vi "Get Message Definition.vi"(8 "error in":errorcluster, 10 "message name":string, 11 "port in":T6 format="%.0x") -> (0 "error out":errorcluster, 2 "message configuration":T1={"name"="", "message type"="BC to RT", "endpoint Tx"={"terminal address"=0, "subaddress"=0}, "endpoint Rx"={"terminal address"=0, "subaddress"=0}, "create timestamp channel"=FALSE, "mode code"=0, "number of words"=0, "parameters"=[]}, 3 "port out":T6 format="%.0x")   [LabVIEW 2020, in "Ballard MIL-STD-1553 Scripting.lvlib"]
uses:
  Ballard MIL-STD-1553 Scripting.lvlib
  <vilib>/NI VeriStand/Custom Device API/Custom Device Item Ref.ctl
  Shared/Message Definition.ctl
  Shared/Message Type.ctl
  Shared/Terminal Endpoint.ctl
  Shared/Address.ctl
  Shared/Parameter Definition.ctl
  Shared/Direction.ctl
  <vilib>/NI VeriStand/Custom Device API/Custom Device API.lvlib
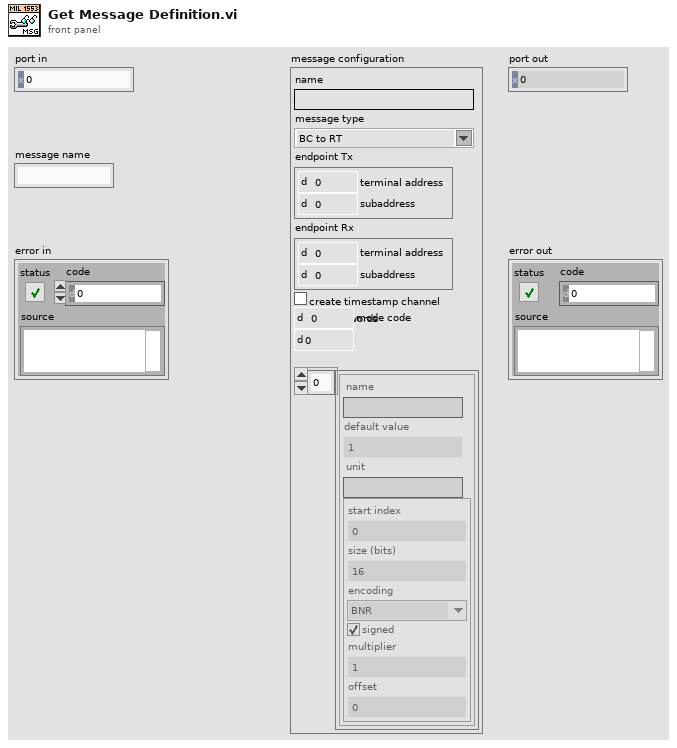
[diagram p1: front panel]
types:
  T1 = typedef "Message Definition.ctl" = cluster{"name":string, "message type":T2, "endpoint Tx":T3, "endpoint Rx":T3, "create timestamp channel":bool, "mode code":u16, "number of words":u16, "parameters":cluster{"name":string, "default value":dbl, "unit":string, "parameter definition":T5}[]}
  T2 = typedef "Message Type.ctl" = string
  T3 = typedef "Terminal Endpoint.ctl" = cluster{"terminal address":T4, "subaddress":T4}
  T4 = typedef "Address.ctl" = u16
  T5 = typedef "Parameter Definition.ctl" = cluster{"start index":i32, "size (bits)":i32, "encoding":enum16{"BNR", "BCD", "Discrete"}, "signed":bool, "multiplier":dbl, "offset":dbl}
  T6 = typedef "Custom Device API.lvlib/Custom Device Item Ref.ctl" = u64
  T7 = typedef "Direction.ctl" = enum16{"Rx", "Tx"}
  T8 = cluster{"name":string, "default value":dbl, "unit":string, "parameter definition":T5}
  T9 = typedef "Custom Device API.lvlib/Custom Device Channel.ctl" = cluster{"Type":T10, "Units":string, "Default Value":dbl, "Faultable":bool, "Scalable":bool}
  T10 = typedef "Custom Device API.lvlib/Custom Device Channel Type.ctl" = enum16{"Input", "Output"}
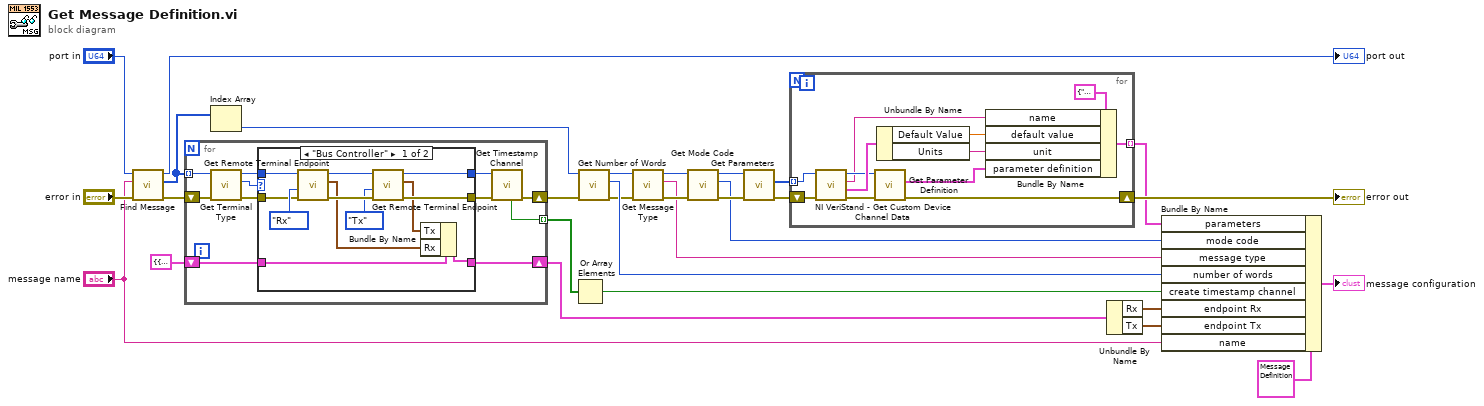
[diagram p0: block diagram]
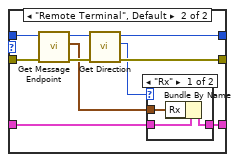
[diagram p2: hidden frame]
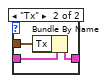
[diagram p3: hidden frame]
diagram:
  n1 = call "Find Message.vi"("error in"="error in", "message name"="message name", "port in"="port in") -> ("error out"=w28:errorcluster, "message refs"=w29:T6[], "port out"=→"port out":T6)  [unwired: 5 in, 1 out]
  n2 = for {
    shift-right: [w39] -> w11
    shift-left: w28 -> [w33]
    tunnel: w29 -> [w34] mode=indexing
    tunnel: [w40] -> w9 mode=indexing
    shift-right: [w35] -> w4
    shift-left: cluster{"Rx":T3, "Tx":T3} {"Rx"={"terminal address"=0, "subaddress"=0}, "Tx"={"terminal address"=0, "subaddress"=0}} -> [w36]
    n3 = call "Get Terminal Type.vi"("error in"=w33, "message in"=w34) -> ("error out"=w31:errorcluster, "terminal type"=w30:enum16{"Bus Controller", "Remote Terminal"}, "message out"=w32:T6)  [unwired: 7 in]
    n4 = case shown="\"Bus Controller\"" w30 {
      tunnel: [w44 w60] -> w38
      tunnel: [w43 w59] -> w37
      tunnel: w36 -> [w49 w56]
      tunnel: [w48 w55] -> w35
      tunnel: w32 -> [w52 w54]
      tunnel: w31 -> [w50 w53]
      frame "Bus Controller" {
        n5 = call "Get Remote Terminal Endpoint.vi"("error in"=w50, "direction"=Direction."Rx", "message in"=w52) -> ("error out"=w47:errorcluster, "remote terminal"=w41:T3, "message out"=w45:T6)  [unwired: 5 in, 1 out]
        n6 = call "Get Remote Terminal Endpoint.vi"("error in"=w47, "direction"=Direction."Tx", "message in"=w45) -> ("error out"=w43:errorcluster, "remote terminal"=w42:T3, "message out"=w44:T6)  [unwired: 5 in, 1 out]
        n7 = Bundle By Name(cluster=w49, "Tx"=w42, "Rx"=w41) -> (w48:cluster{"Rx":T3, "Tx":T3})
      }
      frame "Remote Terminal", Default {
        n8 = call "Get Message Endpoint.vi"("error in"=w53, "message in"=w54) -> ("error out"=w61:errorcluster, "message endpoint"=w57:T3, "message out"=w62:T6)  [unwired: 7 in]
        n9 = call "Get Direction.vi"("error in"=w61, "message in"=w62) -> ("error out"=w59:errorcluster, "direction"=w58:T7, "message out"=w60:T6)  [unwired: 6 in, 1 out]
        n10 = case shown="\"Rx\"" w58 {
          tunnel: w57 -> [w63 w67]
          tunnel: w56 -> [w65 w68]
          tunnel: [w64 w66] -> w55
          frame "Rx" {
            n11 = Bundle By Name(cluster=w65, "Rx"=w63) -> (w64:cluster{"Rx":T3, "Tx":T3})
          }
          frame "Tx" {
            n12 = Bundle By Name(cluster=w68, "Tx"=w67) -> (w66:cluster{"Rx":T3, "Tx":T3})
          }
        }
      }
    }
    n13 = call "Get Timestamp Channel.vi"("error in"=w37, "message in"=w38) -> ("error out"=w39:errorcluster, "found?"=w40:bool)  [unwired: 6 in, 2 out]
  }
  n14 = Index Array(array=w29) -> (element=w12:T6)  [unwired: 1 in]
  n15 = Or Array Elements(Boolean array=w9) -> (logical OR=w8:bool)
  n16 = call "Get Number of Words.vi"("error in"=w11, "message in"=w12) -> ("error out"=w20:errorcluster, "number of words"=w22:u16, "message out"=w17:T6)  [unwired: 7 in]
  n17 = call "Get Message Type.vi"("error in"=w20, "message in"=w17) -> ("error out"=w21:errorcluster, "message type"=w15:T2, "message out"=w18:T6)  [unwired: 6 in, 1 out]
  n18 = call "Get Mode Code.vi"("error in"=w21, "message in"=w18) -> ("error out"=w19:errorcluster, "mode code"=w14:u16, "message out"=w16:T6)  [unwired: 7 in]
  n19 = call "Get Parameters.vi"("error in"=w19, "message in"=w16) -> ("error out"=w24:errorcluster, "parameters"=w23:T6[])  [unwired: 7 in, 1 out]
  n20 = for {
    shift-right: [w80] -> w10
    shift-left: w24 -> [w78]
    tunnel: w23 -> [w76] mode=indexing
    tunnel: [w69] -> w6 mode=indexing
    n21 = call <vilib>:"NI VeriStand - Get Custom Device Channel Data.vi"("error in (no error)"=w78, "Channel Ref in"=w76) -> ("error out"=w75:errorcluster, "Channel"=w79:T9, "Channel Name"=w71:string, "Channel Ref out"=w77:T6)  [unwired: 4 in, 2 out]
    n22 = call "Get Parameter Definition.vi"("error in"=w75, "parameter in"=w77) -> ("error out"=w80:errorcluster, "parameter definition"=w70:T5)  [unwired: 7 in, 1 out]
    n23 = Unbundle By Name(w79) -> ("Default Value"=w73:dbl, "Units"=w72:string)
    n24 = Bundle By Name(cluster=T8 {"name"="", "default value"=1.0, "unit"="", "parameter definition"={"start index"=0, "size (bits)"=16, "encoding"=enum."BNR", "signed"=TRUE, "multiplier"=1.0, "offset"=0.0}} ("definition with default value"), "name"=w71, "default value"=w73, "unit"=w72, "parameter definition"=w70) -> (w69:T8)
  }
  "error out" <- w10
  n25 = Unbundle By Name(w4) -> ("Rx"=w3:T3, "Tx"=w2:T3)
  n26 = Bundle By Name(cluster=T1 {"name"="", "message type"="BC to RT", "endpoint Tx"={"terminal address"=0, "subaddress"=0}, "endpoint Rx"={"terminal address"=0, "subaddress"=0}, "create timestamp channel"=FALSE, "mode code"=0, "number of words"=0, "parameters"=[]} ("message definition"), "parameters"=w6, "mode code"=w14, "message type"=w15, "number of words"=w22, "create timestamp channel"=w8, "endpoint Rx"=w3, "endpoint Tx"=w2, "name"="message name") -> (→"message configuration":T1)
